vi "Serial_Setup.vi"(8 "Error In":errorcluster caption="에러 입력") -> (0 "Error Out":errorcluster caption="에러 출력", 3 "VISA resource name out":refnum<visa-resource-name>)   [LabVIEW 2015]
uses:
  Program Files (x86)/National Instruments/LabVIEW 2015/examples/Instrument IO/Serial/support/Serial - Settings.ctl
  <vilib>/Instr/_visa.llb/VISA Configure Serial Port (Instr).vi
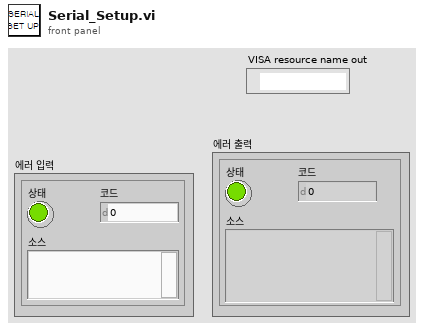
[diagram p1: front panel]
types:
  T1 = typedef "Serial - Settings.ctl" = cluster{"baud rate":u32, "data bits":u16, "parity":enum16{"None", "Odd", "Even", "Mark", "Space"}, "stop bits":u16, "flow control":u16}
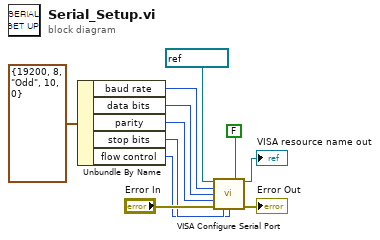
[diagram p0: block diagram]
diagram:
  n1 = Unbundle By Name(T1 {"baud rate"=19200, "data bits"=8, "parity"=enum."Odd", "stop bits"=10, "flow control"=0} ("Serial Settings")) -> ("baud rate"=w6:u32, "data bits"=w5:u16, "parity"=w4:enum16{"None", "Odd", "Even", "Mark", "Space"}, "stop bits"=w3:u16, "flow control"=w2:u16)
  n2 = call-poly "VISA Configure Serial Port"("VISA resource name"=refnum<visa-resource-name> "COM3" ("Port"), "Enable Termination\nChar (T)"=FALSE ("Enable Termination\nChar (T)"), "baud rate (9600)"=w6, "data bits (8)"=w5, "parity (0:none)"=w4, "error in (no error)"="Error In", "stop bits (10: 1 bit)"=w3, "flow control (0:none)"=w2) -> ("VISA resource name out"=→"VISA resource name out":refnum<visa-resource-name>, "error out"=→"Error Out":errorcluster)  [unwired: 1 in, 5 out]
